vi "GA Home Set Prm.vi"(8 "error in (no error)":errorcluster caption="错误输入（无错误）", 10 "pAxisHomePrm":T1, 11 "iAxisNum":i32) -> (0 "error out":errorcluster caption="错误输出", 2 "pAxisHomePrm out":T1, 3 "function return":i32)   [LabVIEW 2024, in "GAS.lvlib"]
doc: "extern \"C\" __declspec(dllimport) int GA_HomeSetPrm(int iAxisNum,TAxisHomePrm *pAxisHomePrm);"
uses:
  GAS.lvlib
  GAS.dll
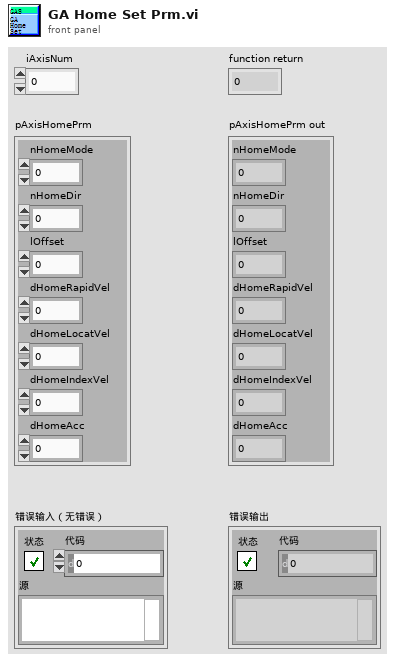
[diagram p1: front panel]
types:
  T1 = cluster{"nHomeMode":i16, "nHomeDir":i16, "lOffset":i32, "dHomeRapidVel":dbl, "dHomeLocatVel":dbl, "dHomeIndexVel":dbl, "dHomeAcc":dbl}
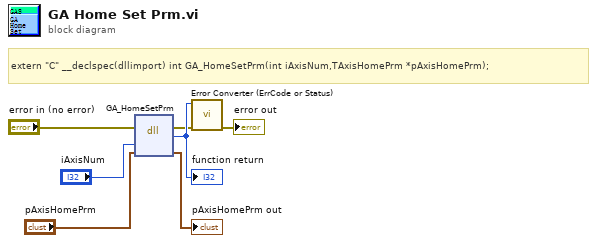
[diagram p0: block diagram]
diagram:
  # "extern \"C\" __declspec(dllimport) int GA_HomeSetPrm(int iAxisNum,TAxisHomePrm *pAxisHomePrm);"
  n1 = dll-call lib="PTH2?abs D实验室软件（勿删）集成测试系统GAS.*" fn="GA_HomeSetPrm"(error in="error in (no error)", "iAxisNum"="iAxisNum", "pAxisHomePrm"="pAxisHomePrm") -> (error out=w2:errorcluster, w7:i32, "pAxisHomePrm"=→"pAxisHomePrm out":T1)  [unwired: 3 in, 1 out]
  "function return" <- w7
  n2 = call "Error Converter (ErrCode or Status).vi"("error in (no error)"=w2, "error code"=w7) -> ("error out"=→"error out":errorcluster)  [unwired: 9 in]
